vi "validate line configuration.vi"(7 "EthernetIP configuration":refnum<class "EIP Tags Configuration.lvclass">, 11 "line in":T1) -> (1 "valid?":bool, 2 "problem":string, 3 "line out":T1)   [LabVIEW 2013, in "EIP Tags editor node.lvclass"]
uses:
  EIP Tags editor node.lvclass
  <vilib>/NI/Tag Bus/tag/tag descriptor.lvclass
  configuration/EIP Tags Configuration.lvclass
  channel/EIP Tags Channel.lvclass
  table line.ctl
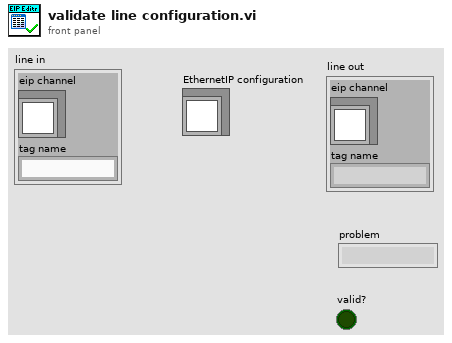
[diagram p1: front panel]
types:
  T1 = typedef "EIP Tags editor node.lvclass/table line.ctl" = cluster{"eip channel":refnum<class "EIP Tags Channel.lvclass">, "tag name":string}
  T2 = typedef "EIP Tags Configuration.lvclass/eip tag definition.ctl" = cluster{"eip tag types":T3, "unique tag name":string, "Number of Elements":u32}
  T3 = typedef "EIP Tags Configuration.lvclass/eip tag types.ctl" = enum16{"SINT", "INT", "DINT", "REAL", "BOOL", "STRING"}
  T4 = typedef "tag bus.lvlib/tag descriptor.lvclass/Data Type.ctl" = enum16{"Double", "Single", "I64", "I32", "I16", "I8", "U64", "U32", "U16", "U8", "Boolean", "String", "Array of Double", "Array of Single", "Array of I64", "Array of I32", "Array of I16", "Array of I8", "Array of U64", "Array of U32", "Array of U16", "Array of U8", "Array of Boolean", "Array of String"}
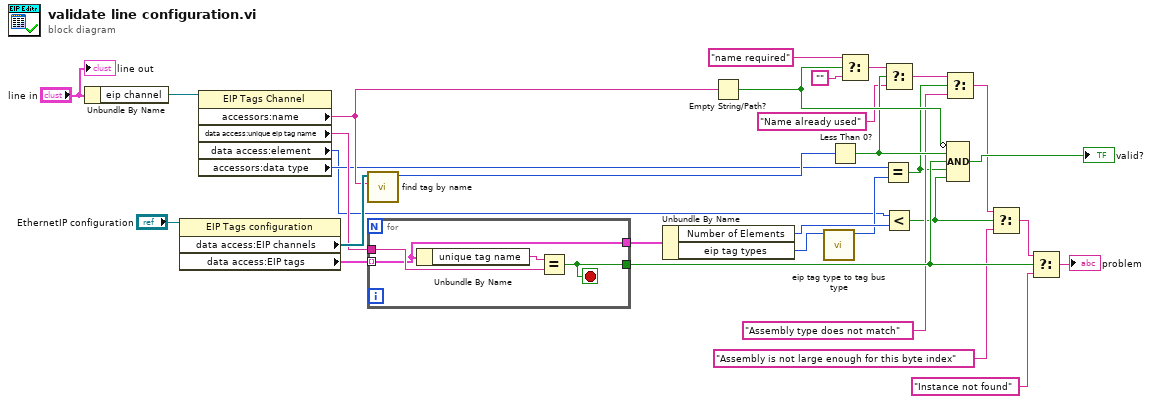
[diagram p0: block diagram]
diagram:
  n1 = Unbundle By Name("line in") -> ("eip channel"=w30:refnum<class "EIP Tags Channel.lvclass">)
  n2 = property class="EIP Tags configuration"(reference="EthernetIP configuration") -> ("data access:EIP channels"=w28:refnum<class "EIP Tags Channel.lvclass">[], "data access:EIP tags"=w24:T2[])  [unwired: 1 in, 2 out]
  n3 = property class="EIP Tags Channel"(reference=w30) -> ("accessors:name"=w27:string, "data access:unique eip tag name"=w18:string, "data access:element"=w1:i32, "accessors:data type"=w4:T4)  [unwired: 1 in, 2 out]
  n4 = call <vilib>:"find tag by name.vi"("name"=w27, "tags in"=w28) -> ("index"=w25:i32)  [unwired: 9 in]
  n5 = for {
    tunnel: w24 -> [w33] mode=indexing
    tunnel: w18 -> [w34]
    tunnel: [w33] -> w12
    tunnel: [w32] -> w16
    stop <- w32 stop-if-true
    n6 = Unbundle By Name(w33) -> ("unique tag name"=w35:string)
    n7 = Equal?(x=w35, y=w34) -> (x = y?=w32:bool)
  }
  n8 = Unbundle By Name(w12) -> ("Number of Elements"=w7:u32, "eip tag types"=w3:T3)
  n9 = Empty String/Path?(string/path=w27) -> (empty?=w23:bool)
  n10 = call "eip tag type to tag bus type.vi"("eip tag types"=w3) -> ("data type"=w2:T4)  [unwired: 10 in]
  n11 = Less Than 0?(x=w25) -> (x < 0?=w22:bool)
  n12 = Select(t="name required", s=w23, f="") -> (s? t:f=w21:string)
  n13 = Equal?(x=w4, y=w2) -> (x = y?=w8:bool)
  n14 = Select(t=w21, s=w22, f="Name already used") -> (s? t:f=w11:string)
  n15 = Less?(x=w1, y=w7) -> (x < y?=w6:bool)
  n16 = Select(t=w11, s=w8, f="Assembly type does not match") -> (s? t:f=w13:string)
  n17 = Compound Arithmetic op=AND(invert w23, w22, w16, w8, w6) -> (→"valid?":bool)
  n18 = Select(t=w13, s=w6, f="Assembly is not large enough for this byte index") -> (s? t:f=w10:string)
  n19 = Select(t=w10, s=w16, f="Instance not found") -> (s? t:f=→"problem":string)
  "line out" <- "line in"
